vi "rqcBob KeyNET Send Data U8.vi"(8 "error in":errorcluster, 10 "Data":u8[](array[numeric]), 11 "rqcBob KeyNET in":T1) -> (0 "error out":errorcluster, 3 "rqcBob KeyNET out":T1)   [LabVIEW 2016]
uses:
  Custom Controls/rqcBob KeyNET control.ctl
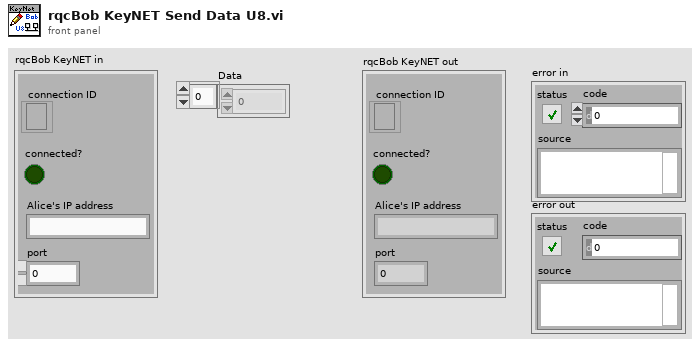
[diagram p1: front panel]
types:
  T1 = typedef "rqcBob KeyNET control.ctl" = cluster{"connection ID":refnum<k5>, "connected?":bool, "Alice's IP address":string, "port":u16}
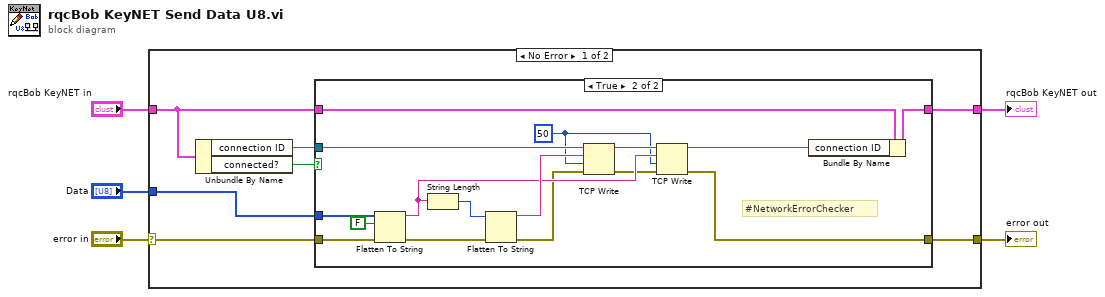
[diagram p0: block diagram]
diagram:
  n1 = case shown="No Error" "error in" {
    selector: "error in" -> [w9 w32]
    tunnel: "rqcBob KeyNET in" -> [w7 w31]
    tunnel: [w8 w32] -> w3
    tunnel: [w6 w31] -> w2
    tunnel: "Data" -> [w10 _]
    frame No Error {
      n2 = Unbundle By Name(w7) -> ("connection ID"=w11:refnum<k5>, "connected?"=w12:bool)
      n3 = case shown="True" w12 {
        tunnel: w11 -> [_ w30]
        tunnel: w10 -> [_ w29]
        tunnel: w9 -> [w14 w28]
        tunnel: [w14 w19] -> w8
        tunnel: [w13 w17] -> w6
        tunnel: w7 -> [w13 w18]
        frame False {
        }
        frame True {
          w15 = 50 ("timeout ms (25000)")
          # "#NetworkErrorChecker"
          n4 = Flatten To String(anything=w29, prepend array or string size? (T)=FALSE, error in (no error)=w28) -> (data string=w23:string, error out=w26:errorcluster)  [unwired: 1 in, 1 out]
          n5 = String Length(string=w23) -> (length=w25:i32)
          n6 = Flatten To String(anything=w25, error in (no error)=w26) -> (data string=w24:string, error out=w22:errorcluster)  [unwired: 2 in, 1 out]
          n7 = TCP Write(connection ID=w30, data in=w24, error in (no error)=w22, 9:w15) -> (connection ID out=w20:refnum<k5>, error out=w21:errorcluster)  [unwired: 1 out]
          n8 = TCP Write(connection ID=w20, data in=w23, error in (no error)=w21, 9:w15) -> (connection ID out=w16:refnum<k5>, error out=w19:errorcluster)  [unwired: 1 out]
          n9 = Bundle By Name(cluster=w18, "connection ID"=w16) -> (w17:T1)
        }
      }
    }
    frame Error {
    }
  }
  "error out" <- w3
  "rqcBob KeyNET out" <- w2
